vi "Init.vi"(8 "error in (no error)":errorcluster, 10 "serial port":refnum<visa-resource-name>, 11 "Serial in":refnum<class "Serial.lvclass">) -> (0 "error out":errorcluster, 3 "Serial out":refnum<class "Serial.lvclass">)   [LabVIEW 2014, in "Serial.lvclass"]
uses:
  Serial.lvclass
  Serial.lvclass/Serial.ctl
  <vilib>/Instr/_visa.llb/VISA Configure Serial Port (Instr).vi
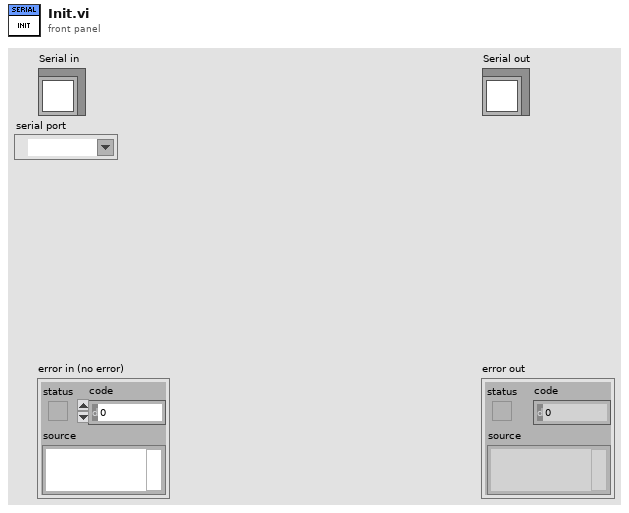
[diagram p1: front panel]
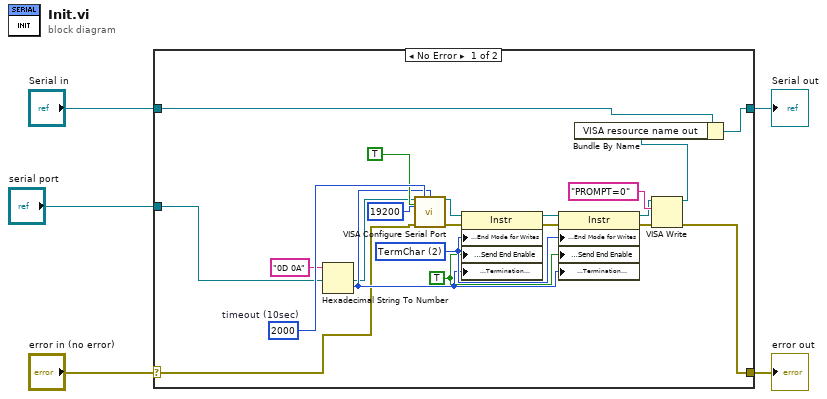
[diagram p0: block diagram]
diagram:
  n1 = case shown="No Error" "error in (no error)" {
    selector: "error in (no error)" -> [w6 w27]
    tunnel: [w7 w27] -> w4
    tunnel: [w9 w26] -> w2
    tunnel: "Serial in" -> [w10 w26]
    tunnel: "serial port" -> [w11 _]
    frame No Error {
      w17 = TRUE ("Message Based Settings:Send End Enable")
      w18 = u16 2 items=["None", "LastBit", "TermChar", "Break"] ("Serial Settings:Serial End Mode for Writes")
      w25 = u32 2000  # timeout (10sec)
      n2 = Hexadecimal String To Number(string="0D 0A") -> (number=w16:u32)  [unwired: 2 in, 1 out]
      n3 = call-poly "VISA Configure Serial Port"("VISA resource name"=w11, "timeout (10sec)"=w25, "termination char\n(0xA = '\\n' = LF)"=w16, "Enable Termination\nChar (T)"=TRUE ("Enable Termination\nChar (T)"), "baud rate (9600)"=u32 19200, "error in (no error)"=w6) -> ("VISA resource name out"=w22:refnum<visa-resource-name>, "error out"=w21:errorcluster)  [unwired: 4 in, 4 out]
      n4 = property class="Instr"(reference=w22, error in=w21, "Serial Settings:End Mode for Writes"=w18, "Message Based Settings:Send End Enable"=w17, "Message Based Settings:Termination Character"=w16) -> (reference out=w20:refnum<visa-resource-name>, error out=w19:errorcluster)
      n5 = property class="Instr"(reference=w20, error in=w19, "Serial Settings:End Mode for Writes"=w18, "Message Based Settings:Send End Enable"=w17, "Message Based Settings:Termination Character"=w16) -> (reference out=w13:refnum<visa-resource-name>, error out=w12:errorcluster)
      n6 = VISA Write(VISA resource name=w13, write buffer="PROMPT=0", error in (no error)=w12) -> (VISA resource name out=w8:refnum<visa-resource-name>, error out=w7:errorcluster)  [unwired: 1 out]
      n7 = Bundle By Name(cluster=w10, "VISA resource name out"=w8) -> (w9:refnum<class "Serial.lvclass">)
    }
    frame Error {
    }
  }
  "error out" <- w4
  "Serial out" <- w2
